vi "Stop_Tasks.vi"(8 "error in (no error)":errorcluster, 11 "Task cluster In":T1) -> (0 "error out":errorcluster, 3 "Task cluster Out":T1)   [LabVIEW 2018, in "Motor_ReadAng.lvlib"]
doc: "Stops all tasks reference from cluster in"
uses:
  Motor_ReadAng.lvlib
  Task cluster.ctl
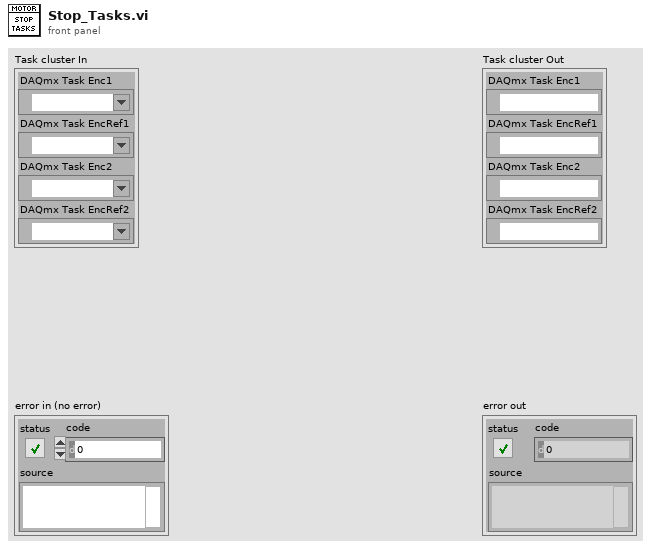
[diagram p1: front panel]
types:
  T1 = typedef "Motor_ReadAng.lvlib/Task cluster.ctl" = cluster{"DAQmx Task Enc1":refnum<k21>, "DAQmx Task EncRef1":refnum<k21>, "DAQmx Task Enc2":refnum<k21>, "DAQmx Task EncRef2":refnum<k21>}
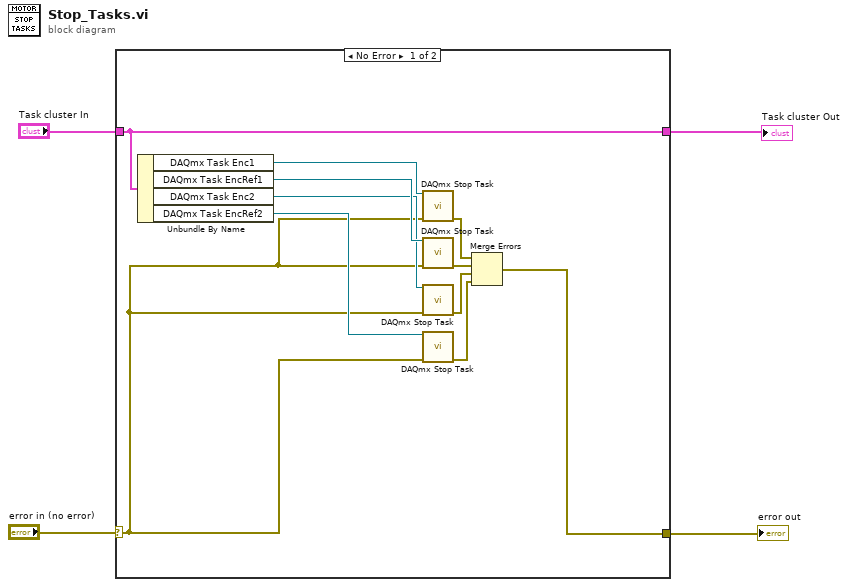
[diagram p0: block diagram]
diagram:
  n1 = case shown="No Error" "error in (no error)" {
    selector: "error in (no error)" -> [w11 w17]
    tunnel: [w10 w17] -> w3
    tunnel: "Task cluster In" -> [w5 w16]
    tunnel: [w5 w16] -> w1
    frame No Error {
      n2 = Unbundle By Name(w5) -> ("DAQmx Task Enc1"=w15:refnum<k21>, "DAQmx Task EncRef1"=w14:refnum<k21>, "DAQmx Task Enc2"=w13:refnum<k21>, "DAQmx Task EncRef2"=w12:refnum<k21>)
      n3 = call <vilib>:"DAQmx Stop Task.vi"("task/channels in"=w15, "error in"=w11) -> ("error out"=w9:errorcluster)  [unwired: 12 in, 1 out]
      n4 = call <vilib>:"DAQmx Stop Task.vi"("task/channels in"=w14, "error in"=w11) -> ("error out"=w8:errorcluster)  [unwired: 12 in, 1 out]
      n5 = call <vilib>:"DAQmx Stop Task.vi"("task/channels in"=w13, "error in"=w11) -> ("error out"=w7:errorcluster)  [unwired: 12 in, 1 out]
      n6 = call <vilib>:"DAQmx Stop Task.vi"("task/channels in"=w12, "error in"=w11) -> ("error out"=w6:errorcluster)  [unwired: 12 in, 1 out]
      n7 = Merge Errors(w9, w8, w7, w6) -> (w10:errorcluster)
    }
    frame Error {
    }
  }
  "error out" <- w3
  "Task cluster Out" <- w1
